vi "DQMH System Message - Add to Run-Time Menu.vi"(9 "Module Descriptor":string, 10 "Module Directory Path":path) -> (1 "Payload":variant, 2 "Identifier":string="Add to Run-Time Menu", 5 "Source":T1)   [LabVIEW 2014, in "hse-dqmh.lvlib"]
uses:
  hse-dqmh.lvlib
  Controls/System Message Source.ctl
  Controls/System Message Framework Identifiers.ctl
  Controls/System Message - Add to Run-Time Menu - Argument--cluster.ctl
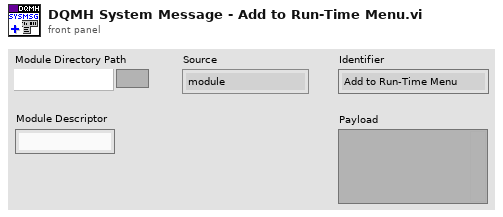
[diagram p1: front panel]
types:
  T1 = typedef "hse-dqmh.lvlib/System Message Source.ctl" = enum16{"module", "application", "network"}
  T2 = typedef "hse-dqmh.lvlib/System Message - Add to Run-Time Menu - Argument--cluster.ctl" = cluster{"Module Directory Path":path, "Module Descriptor":string}
  T3 = typedef "hse-dqmh.lvlib/System Message Framework Identifiers.ctl" = enum16{"Add to Run-Time Menu", "Ready for Display", "Removed from Subpanel"}
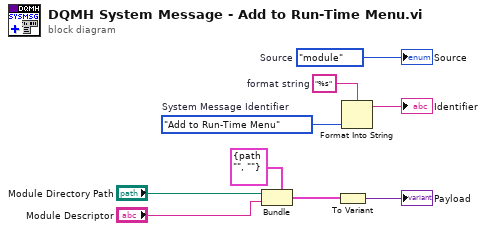
[diagram p0: block diagram]
diagram:
  w5 = "%s"  # format string
  w7 = System_Message_Framework_Identifiers."Add to Run-Time Menu"  # System Message Identifier
  w9 = System_Message_Source."module"  # Source
  n1 = Bundle(cluster=T2 {"Module Directory Path"=path "", "Module Descriptor"=""}, "Module Directory Path"="Module Directory Path", "Module Descriptor"="Module Descriptor") -> (w2:T2)
  n2 = To Variant(anything=w2) -> (Variant=→"Payload":variant)
  n3 = Format Into String(format string=w5, w7) -> (resulting string=→"Identifier":string)  [unwired: 2 in, 1 out]
  "Source" <- w9
